vi "Inspect HDI Pad Groups.vi"(7 "Console Log in":refnum<class "Console Log.lvclass">, 8 "error in":errorcluster, 10 "Module Data In":T1={"TBM-TBM"={"Fiducial Image"={"Image Position"=refnum, "Image Reference"=refnum, "Field of View"={"x(mm)"=0.0, "y(mm)"=0.0}}, "Fiducials"=[]}, "TBM-HDI"={"Fiducial Image"={"Image Position"=refnum, "Image Reference"=refnum, "Field of View"={"x(mm)"=0.0, "y(mm)"=0.0}}, "Fiducials"=[]}, "Address Pads"={"Fiducial Image"={"Image Position"=refnum, "Image Reference"=refnum, "Field of View"={"x(mm)"=0.0, "y(mm)"=0.0}}, "Fiducials"=[]}, "HDI Bond Pad References"=[], "BBM Bond Pad References"=[], "HV-HDI"={"Fiducial Image"={"Image Position"=refnum, "Image Reference"=refnum, "Field of View"={"x(mm)"=0.0, "y(mm)"=0.0}}, "Selected Fiducial"={"Fiducial Image Coordinate"=refnum, "Fiducial Source"=enum."Pattern Recognition"}, "fiducial name"=""}, "HV-BBM"={"Fiducial Image"={"Image Position"=refnum, "Image Reference"=refnum, "Field of View"={"x(mm)"=0.0, "y(mm)"=0.0}}, "Selected Fiducial"={"Fiducial Image Coordinate"=refnum, "Fiducial Source"=enum."Pattern Recognition"}, "fiducial name"=""}, "Chuck"=0, "Slot"=0, "Potting Selection"={"HDI Bond Pads"=[TRUE, TRUE, TRUE, TRUE, TRUE, TRUE, TRUE, TRUE, TRUE, TRUE, TRUE, TRUE, TRUE, TRUE, TRUE, TRUE], "BBM Bond Pads"=[TRUE, TRUE, TRUE, TRUE, TRUE, TRUE, TRUE, TRUE, TRUE, TRUE, TRUE, TRUE, TRUE, TRUE, TRUE, TRUE], "TBM Inner"={"Top"=TRUE, "Left"=TRUE, "Bottom"=TRUE, "Right"=TRUE}, "TBM Outer"={"Top"=TRUE, "Left"=TRUE, "Bottom"=TRUE, "Right"=TRUE}, "Address Pads"={"Top"=TRUE, "Bottom"=TRUE}, "High Voltage"={"HDI"=TRUE, "BBM"=TRUE}}}, 11 "Potting Procedure in":refnum<class "Potting Procedure.lvclass">) -> (0 "error out":errorcluster, 2 "Module Data Out":T1={"TBM-TBM"={"Fiducial Image"={"Image Position"=refnum, "Image Reference"=refnum, "Field of View"={"x(mm)"=0.0, "y(mm)"=0.0}}, "Fiducials"=[]}, "TBM-HDI"={"Fiducial Image"={"Image Position"=refnum, "Image Reference"=refnum, "Field of View"={"x(mm)"=0.0, "y(mm)"=0.0}}, "Fiducials"=[]}, "Address Pads"={"Fiducial Image"={"Image Position"=refnum, "Image Reference"=refnum, "Field of View"={"x(mm)"=0.0, "y(mm)"=0.0}}, "Fiducials"=[]}, "HDI Bond Pad References"=[], "BBM Bond Pad References"=[], "HV-HDI"={"Fiducial Image"={"Image Position"=refnum, "Image Reference"=refnum, "Field of View"={"x(mm)"=0.0, "y(mm)"=0.0}}, "Selected Fiducial"={"Fiducial Image Coordinate"=refnum, "Fiducial Source"=enum."Pattern Recognition"}, "fiducial name"=""}, "HV-BBM"={"Fiducial Image"={"Image Position"=refnum, "Image Reference"=refnum, "Field of View"={"x(mm)"=0.0, "y(mm)"=0.0}}, "Selected Fiducial"={"Fiducial Image Coordinate"=refnum, "Fiducial Source"=enum."Pattern Recognition"}, "fiducial name"=""}, "Chuck"=0, "Slot"=0, "Potting Selection"={"HDI Bond Pads"=[TRUE, TRUE, TRUE, TRUE, TRUE, TRUE, TRUE, TRUE, TRUE, TRUE, TRUE, TRUE, TRUE, TRUE, TRUE, TRUE], "BBM Bond Pads"=[TRUE, TRUE, TRUE, TRUE, TRUE, TRUE, TRUE, TRUE, TRUE, TRUE, TRUE, TRUE, TRUE, TRUE, TRUE, TRUE], "TBM Inner"={"Top"=TRUE, "Left"=TRUE, "Bottom"=TRUE, "Right"=TRUE}, "TBM Outer"={"Top"=TRUE, "Left"=TRUE, "Bottom"=TRUE, "Right"=TRUE}, "Address Pads"={"Top"=TRUE, "Bottom"=TRUE}, "High Voltage"={"HDI"=TRUE, "BBM"=TRUE}}}, 3 "Potting Procedure out":refnum<class "Potting Procedure.lvclass">, 5 "Console Log out":refnum<class "Console Log.lvclass">)   [LabVIEW 2017, in "Potting Procedure.lvclass"]
uses:
  Potting Procedure.lvclass
  Shared Components/Vec3d Class/Vec3d Class.lvclass
  <vilib>/vision/Image Controls.llb/IMAQ Image.ctl
  Shared Components/Utils/Type Definitions/Physical Image.ctl
  Shared Components/Utils/Type Definitions/Fiducial with Source.ctl
  Shared Components/Utils/Type Definitions/Fiducial Image.ctl
  Shared Components/WorkTable Class/WorkTable Class.lvclass
  Shared Components/Gantry Class/Gantry Class.lvclass
  Application Utilities/Console Log/Console Log.lvclass
  Shared Components/Config Manager Class/Config Manager Class.lvclass
  Shared Components/Config Manager Class/Read Geometry Definition 3D.vi
  Shared Components/Config Manager Class/Type Definitions/Part Type.ctl
  Shared Components/Config Manager Class/Type Definitions/Camera Enum.ctl
  Shared Components/Utils/Type Definitions/Multi-Fiducial Image.ctl
  Type Definitions/Inspect Modules - Module.ctl
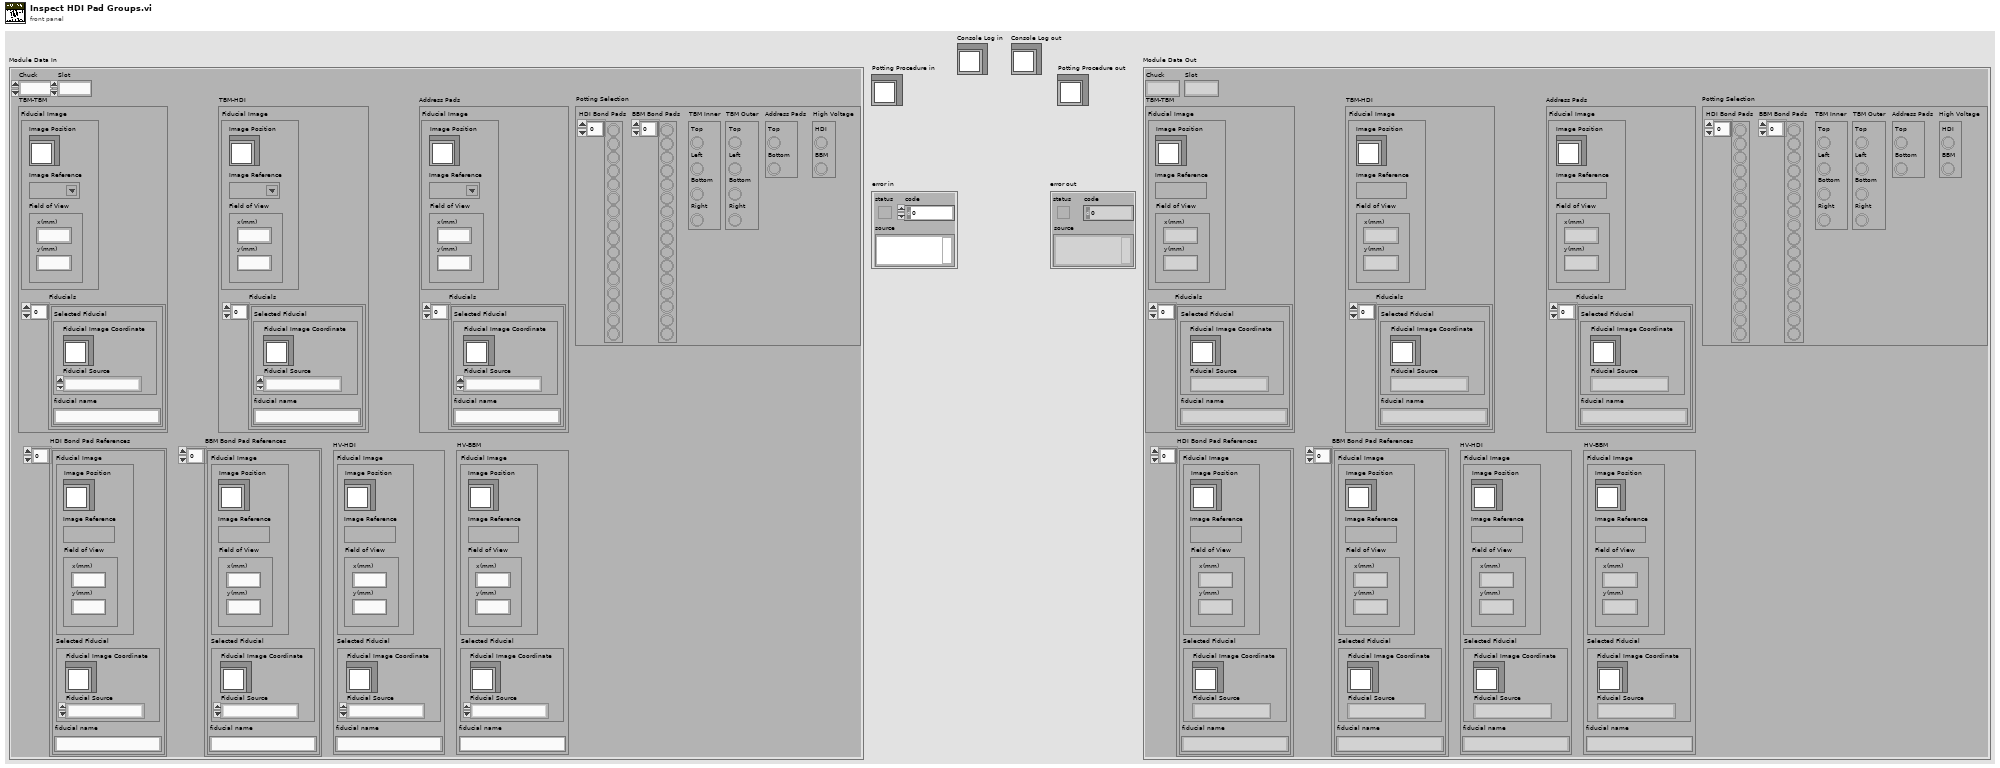
[diagram p1: front panel]
types:
  T1 = typedef "Inspect Modules - Module.ctl" = cluster{"TBM-TBM":T2, "TBM-HDI":T2, "Address Pads":T2, "HDI Bond Pad References":T6[], "BBM Bond Pad References":T6[], "HV-HDI":T6, "HV-BBM":T6, "Chuck":i32, "Slot":i32, "Potting Selection":cluster{"HDI Bond Pads":bool[], "BBM Bond Pads":bool[], "TBM Inner":cluster{"Top":bool, "Left":bool, "Bottom":bool, "Right":bool}, "TBM Outer":cluster{"Top":bool, "Left":bool, "Bottom":bool, "Right":bool}, "Address Pads":cluster{"Top":bool, "Bottom":bool}, "High Voltage":cluster{"HDI":bool, "BBM":bool}}}
  T2 = typedef "Multi-Fiducial Image.ctl" = cluster{"Fiducial Image":T3, "Fiducials":cluster{"Selected Fiducial":T5, "fiducial name":string}[]}
  T3 = typedef "Physical Image.ctl" = cluster{"Image Position":refnum<class "Vec3d Class.lvclass">, "Image Reference":T4, "Field of View":cluster{"x(mm)":dbl, "y(mm)":dbl}}
  T4 = typedef "IMAQ Image.ctl" = refnum<image>
  T5 = typedef "Fiducial with Source.ctl" = cluster{"Fiducial Image Coordinate":refnum<class "Vec3d Class.lvclass">, "Fiducial Source":enum16{"Pattern Recognition", "User", "Error", "Default"}}
  T6 = typedef "Fiducial Image.ctl" = cluster{"Fiducial Image":T3, "Selected Fiducial":T5, "fiducial name":string}
  T7 = typedef "Camera Enum.ctl" = enum16{"GANTRY HEAD", "NEEDLE CALIBRATION X", "NEEDLE CALIBRATION Y"}
  T8 = typedef "Part Type.ctl" = enum16{"BBM", "HDI", "BARE HDI", "GLUERESERVOIR", "STAMP_1", "STAMP_2", "STAMP_3", "STAMP_4", "STAMP_5", "WEIGHT_1", "WEIGHT_2", "WEIGHT_3", "WEIGHT_4", "WEIGHT_5", "WEIGHT_6", "WEIGHT_7", "WEIGHT_8", "PICKER_TOOL", "GRABER_TOOL"}
  T9 = enum16{"Pattern Recognition", "User", "Error", "Default"}
  T10 = typedef "Worktable_Module Slot.ctl" = cluster{"Slot State":enum16{"Empty", "Bare HDI", "Unglued", "Stamped", "PartOnTop", "Weighted", "Unpotted", "Potted"}, "BBM Type":enum16{"None", "BBM", "GlassSlide"}, "HDI Type":enum16{"None", "HDI", "Polyimide"}, "Vacuum Channel":u8, "Location/Orientation BBM":T11, "Location/Orientation HDI":T11, "S/N":string}
  T11 = typedef "Position_Orientation.ctl" = cluster{"Center":refnum<class "Vec3d Class.lvclass">, "Orientation":refnum<class "Orient3d Class.lvclass">}
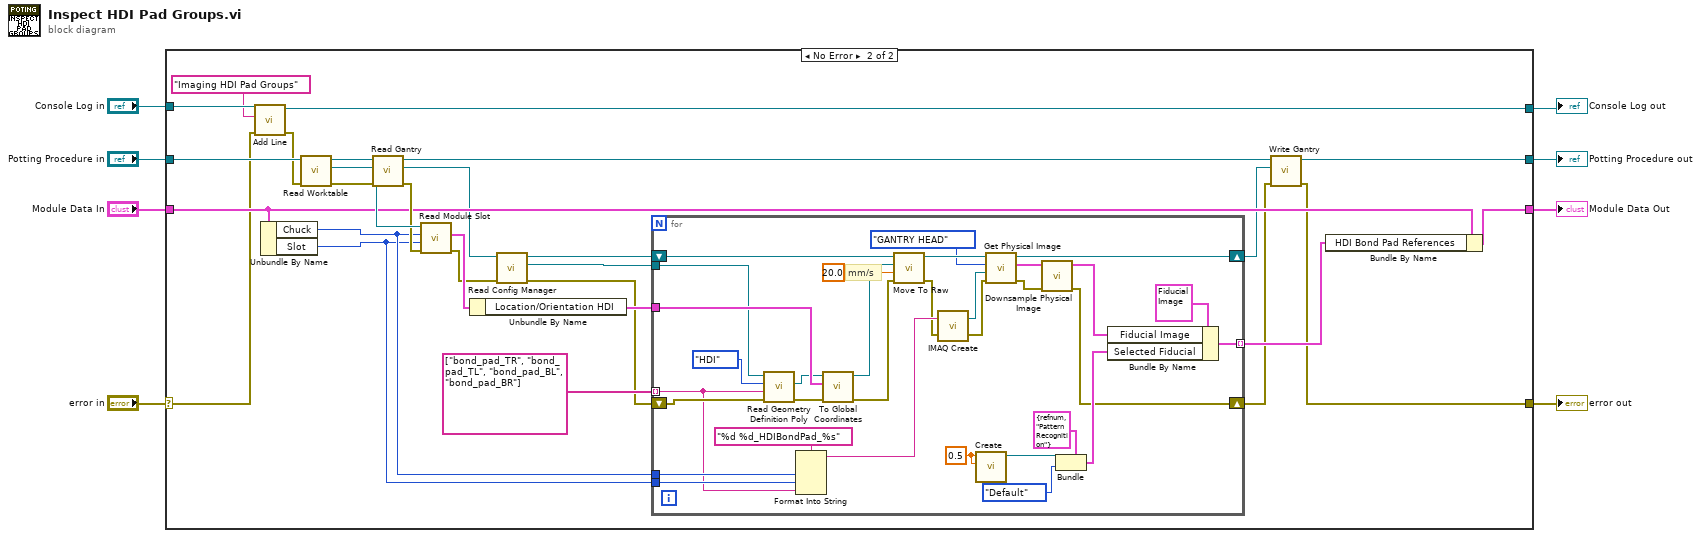
[diagram p0: block diagram]
diagram:
  n1 = case shown="No Error" "error in" {
    selector: "error in" -> [w11 w14]
    tunnel: [w11 w24] -> w7
    tunnel: [w12 w26] -> w5
    tunnel: "Potting Procedure in" -> [w12 w40]
    tunnel: "Module Data In" -> [w10 w31]
    tunnel: [w10 w30] -> w1
    tunnel: "Console Log in" -> [w9 w23]
    tunnel: [w9 w22] -> w3
    frame Error {
    }
    frame No Error {
      n2 = call "Add Line.vi"("error in"=w14, "String"="Imaging HDI Pad Groups", "Console Log in"=w23) -> ("error out"=w13:errorcluster, "Console Log out"=w22:refnum<class "Console Log.lvclass">)  [unwired: 7 in]
      n3 = Unbundle By Name(w31) -> ("Chuck"=w33:i32, "Slot"=w32:i32)
      n4 = call-dynamic "Read Worktable.vi"("error in"=w13, "Potting Procedure in"=w40) -> ("error out"=w38:errorcluster, "WorkTable out"=w37:refnum<class "WorkTable Class.lvclass">, "Potting Procedure out"=w39:refnum<class "Potting Procedure.lvclass">)  [unwired: 7 in]
      n5 = call-dynamic "Read Gantry.vi"("error in (no error)"=w38, "Potting Procedure in"=w39) -> ("error out"=w36:errorcluster, "Gantry"=w20:refnum<class "Gantry Class.lvclass">, "Potting Procedure out"=w27:refnum<class "Potting Procedure.lvclass">)  [unwired: 7 in]
      n6 = call-dynamic "Read Module Slot.vi"("error in"=w36, "slot"=w32, "chuck"=w33, "WorkTable in"=w37) -> ("error out"=w18:errorcluster, "Module Slot"=w35:T10)  [unwired: 5 in, 1 out]
      n7 = Unbundle By Name(w35) -> ("Location/Orientation HDI"=w34:T11)
      n8 = call-dynamic "Read Config Manager.vi"("error in"=w18, "Gantry in"=w20) -> ("error out"=w15:errorcluster, "Config Manager"=w16:refnum<class "Config Manager Class.lvclass">, "Gantry out"=w19:refnum<class "Gantry Class.lvclass">)  [unwired: 7 in]
      n9 = for {
        tunnel: string[] ["bond_pad_TR", "bond_pad_TL", "bond_pad_BL", "bond_pad_BR"] -> [w48] mode=indexing
        tunnel: w34 -> [w72]
        shift-right: [w42] -> w25
        shift-left: w15 -> [w49]
        tunnel: w33 -> [w65]
        tunnel: w32 -> [w64]
        shift-right: [w59] -> w28
        shift-left: w19 -> [w71]
        tunnel: [w52] -> w29 mode=indexing
        tunnel: w16 -> [w51]
        w54 = 0.5 ("X")
        # "mm/s"
        n10 = call-poly "Read Geometry Definition Poly.vi"("error in"=w49, "Feature"=w48, "Part Type"=Part_Type."HDI", "Config Manager in"=w51) -> ("error out"=w46:errorcluster, "Feature Coordinates"=w47:refnum<class "Vec3d Class.lvclass">)  [unwired: 5 in, 1 out]
        n11 = Format Into String(format string="%d %d_HDIBondPad_%s", w65, w64, w48) -> (resulting string=w63:string)  [unwired: 2 in, 1 out]
        n12 = call "To Global Coordinates.vi"("error in"=w46, "Center/Orientation"=w72, "Local Coordinates"=w47) -> ("error out"=w68:errorcluster, "Global Coordinates"=w70:refnum<class "Vec3d Class.lvclass">)  [unwired: 7 in]
        n13 = call-dynamic "Move To Raw.vi"("error in"=w68, "Speed"=20.0, "Destination"=w70, "Gantry in"=w71) -> ("error out"=w62:errorcluster, "Gantry out"=w67:refnum<class "Gantry Class.lvclass">)  [unwired: 6 in]
        n14 = call "IMAQ Create"("Image Name"=w63, "error in (no error)"=w62) -> ("New Image"=w60:T4, "error out"=w61:errorcluster)  [unwired: 3 in]
        n15 = call "Create.vi"("Y"=w54, "X"=w54) -> ("Vec3d Class out"=w55:refnum<class "Vec3d Class.lvclass">)  [unwired: 8 in, 1 out]
        n16 = call-dynamic "Get Physical Image.vi"("error in"=w61, "Image In"=w60, "Camera Name"=Camera_Enum."GANTRY HEAD", "Gantry in"=w67) -> ("error out"=w43:errorcluster, "Physical Image"=w44:T3, "Gantry out"=w59:refnum<class "Gantry Class.lvclass">)  [unwired: 5 in]
        n17 = call "Downsample Physical Image.vi"("error in"=w43, "Physical Image In"=w44) -> ("error out"=w42:errorcluster, "Physical Image Out"=w41:T3)  [unwired: 8 in]
        n18 = Bundle(cluster=T5 {"Fiducial Image Coordinate"=refnum, "Fiducial Source"=enum."Pattern Recognition"} ("Selected Fiducial"), "Fiducial Image Coordinate"=w55, "Fiducial Source"=T9."Default") -> (w56:T5)
        n19 = Bundle By Name(cluster=T6 {"Fiducial Image"={"Image Position"=refnum, "Image Reference"=refnum, "Field of View"={"x(mm)"=0.0, "y(mm)"=0.0}}, "Selected Fiducial"={"Fiducial Image Coordinate"=refnum, "Fiducial Source"=enum."Pattern Recognition"}, "fiducial name"=""} ("Fiducial Image"), "Fiducial Image"=w41, "Selected Fiducial"=w56) -> (w52:T6)
      }
      n20 = call-dynamic "Write Gantry.vi"("error in (no error)"=w25, "Gantry"=w28, "Potting Procedure in"=w27) -> ("error out"=w24:errorcluster, "Potting Procedure out"=w26:refnum<class "Potting Procedure.lvclass">)  [unwired: 7 in]
      n21 = Bundle By Name(cluster=w31, "HDI Bond Pad References"=w29) -> (w30:T1)
    }
  }
  "error out" <- w7
  "Potting Procedure out" <- w5
  "Console Log out" <- w3
  "Module Data Out" <- w1
